vi "5.3.vi"() -> ()   [LabVIEW 2017]
uses:
  <vilib>/Utility/file.llb/Write Delimited Spreadsheet (DBL).vi
  <vilib>/Utility/file.llb/Read Delimited Spreadsheet (DBL).vi
  <vilib>/measure/NI_MABase.lvlib
panel:
  out "原波形":waveform(dbl)(graph)
  out "电子表格":cluster{i32, "Numeric":dbl, dbl[][]}(graph)
  out "二进制文件":waveform(dbl)(graph)
  out "文本文件":cluster{i32, dbl, dbl[][]}(graph)
  # "任务三"
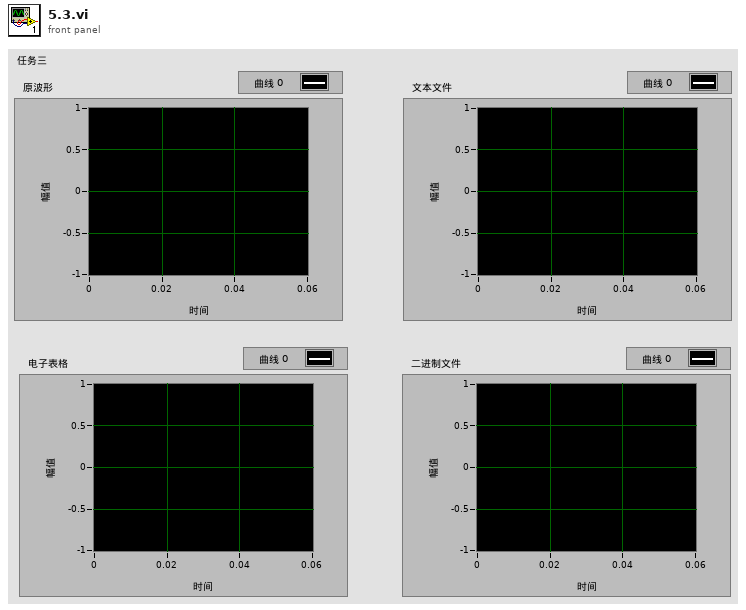
[diagram p1: front panel]
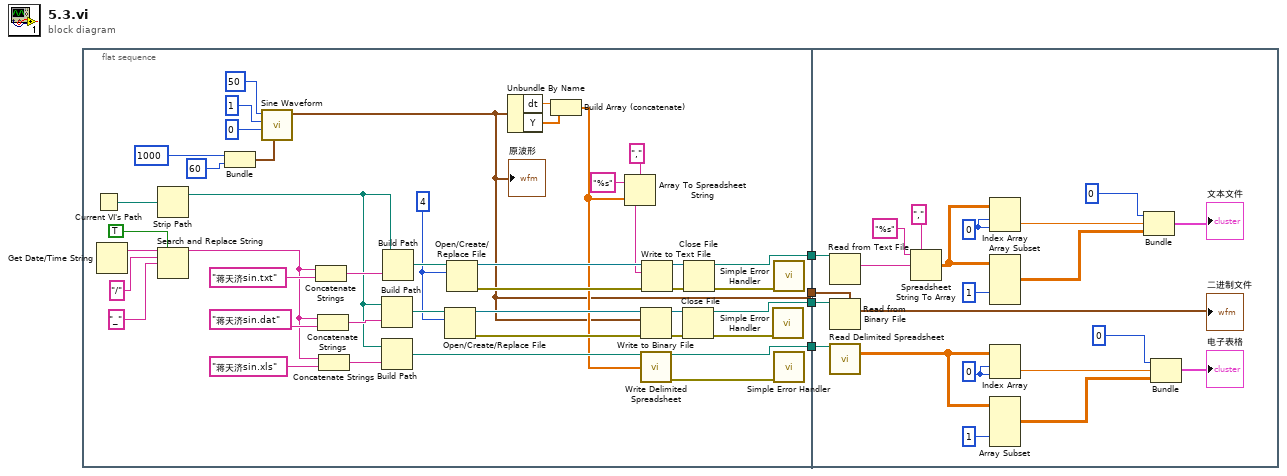
[diagram p0: block diagram]
diagram:
  n1 = flat-sequence {
    tunnel: [w8] -> w4
    tunnel: [w7] -> w3
    tunnel: [w6] -> w2
    tunnel: [w5] -> w1
    tunnel: w4 -> [w70]
    tunnel: w3 -> [w69]
    tunnel: w2 -> [w68]
    tunnel: w1 -> [w57]
    frame #0 {
      w22 = 4
      n2 = Current VI's Path() -> (path=w37:path)
      n3 = Get Date/Time String() -> (date string=w15:string)  [unwired: 3 in, 1 out]
      n4 = Strip Path(path=w37) -> (stripped path=w30:path)  [unwired: 1 out]
      n5 = Search and Replace String(replace all?=TRUE, input string=w15, search string="/" ("搜索字符串"), replace string="_" ("搜索字符串")) -> (result string=w12:string)  [unwired: 4 in, 3 out]
      n6 = Bundle(1000, 60) -> (w38:cluster{i32, i32})  [unwired: 1 in]
      n7 = call <vilib>:"Sine Waveform.vi"("sampling info"=w38, "phase"=0, "amplitude"=1, "frequency"=50) -> ("signal out"=w5:waveform(dbl))  [unwired: 6 in, 1 out]
      "原波形" <- w5
      n8 = Concatenate Strings(w12, "蒋天济sin.txt") -> (w33:string)
      n9 = Concatenate Strings(w12, "蒋天济sin.dat") -> (w32:string)
      n10 = Concatenate Strings(w12, "蒋天济sin.xls") -> (w31:string)
      n11 = Build Path(base path=w30, name or relative path=w32) -> (appended path=w29:path)
      n12 = Build Path(base path=w30, name or relative path=w31) -> (appended path=w21:path)
      n13 = Build Path(base path=w30, name or relative path=w33) -> (appended path=w23:path)
      n14 = Open/Create/Replace File(file path (use dialog)=w29, operation (0:open)=w22) -> (refnum out=w47:refnum<file>, error out=w48:errorcluster)  [unwired: 4 in, 1 out]
      n15 = Open/Create/Replace File(file path (use dialog)=w23, operation (0:open)=w22) -> (refnum out=w27:refnum<file>, error out=w28:errorcluster)  [unwired: 4 in, 1 out]
      n16 = Unbundle By Name(w5) -> ("dt"=w9:dbl, "Y"=w19:dbl[])
      n17 = Build Array (concatenate)(w9, w19) -> (w10:dbl[])
      n18 = Array To Spreadsheet String(delimiter (Tab)="," ("分隔符(Tab)"), array=w10, 3:"%s" ("格式字符串")) -> (spreadsheet string=w16:string)
      n19 = Write to Binary File(file (use dialog)=w47, data=w5, error in=w48) -> (refnum out=w46:refnum<file>, error out=w45:errorcluster)  [unwired: 3 in, 1 out]
      n20 = call-poly <vilib>:"Write Delimited Spreadsheet.vi"("file path (dialog if empty)"=w21, "1D data"=w10) -> ("new file path (Not A Path if cancelled)"=w6:path, "error out"=w20:errorcluster)  [unwired: 12 in]
      n21 = Write to Text File(file (use dialog)=w27, text=w16, error in=w28) -> (refnum out=w26:refnum<file>, error out=w25:errorcluster)  [unwired: 1 in, 1 out]
      n22 = Close File(refnum=w46, error in=w45) -> (path=w7:path, error out=w41:errorcluster)
      n23 = Close File(refnum=w26, error in=w25) -> (path=w8:path, error out=w24:errorcluster)
      n24 = call <vilib>:"Simple Error Handler.vi"("error in (no error)"=w41) -> ()  [unwired: 4 in, 5 out]
      n25 = call <vilib>:"Simple Error Handler.vi"("error in (no error)"=w24) -> ()  [unwired: 4 in, 5 out]
      n26 = call <vilib>:"Simple Error Handler.vi"("error in (no error)"=w20) -> ()  [unwired: 4 in, 5 out]
    }
    frame #1 {
      w52 = 0 ("索引 (行)")
      w60 = 0 ("索引 (行)")
      n27 = Read from Text File(file (use dialog)=w70) -> (text=w67:string)  [unwired: 3 in, 3 out]
      n28 = Read from Binary File(5:w57, 11:w69) -> (2:→"二进制文件":waveform(dbl))  [unwired: 4 in, 3 out]
      n29 = call-poly <vilib>:"Read Delimited Spreadsheet.vi"("file path (dialog if empty)"=w68) -> ("all rows"=w50:dbl[][])  [unwired: 9 in, 5 out]
      n30 = Spreadsheet String To Array(delimiter (Tab)="," ("分隔符(Tab)"), format string="%s" ("格式字符串"), spreadsheet string=w67) -> (array=w64:dbl[][])  [unwired: 1 in]
      n31 = Index Array(array=w64, index (row)=w60, index (col)=w60) -> (element=w63:dbl)
      n32 = Array Subset(array=w64, index (col)=1 ("索引")) -> (w62:dbl[][])  [unwired: 3 in]
      n33 = Index Array(array=w50, index (row)=w52, index (col)=w52) -> (element=w55:dbl)
      n34 = Array Subset(array=w50, index (col)=1 ("索引")) -> (w54:dbl[][])  [unwired: 3 in]
      n35 = Bundle(0, w63, w62) -> (→"文本文件":cluster{i32, dbl, dbl[][]})  [unwired: 1 in]
      n36 = Bundle(0, "Numeric"=w55, w54) -> (→"电子表格":cluster{i32, "Numeric":dbl, dbl[][]})  [unwired: 1 in]
    }
  }
